vi "data_store.vi"(9 "Action":enum16{"set values", "get values"}(ring), 11 "number of elements":i32=10000) -> (1 "Variant":variant, 2 "array items":cluster{"name":string, "address":string}[](array[cluster]), 3 "names":string[](array[string]))   [LabVIEW 2018]
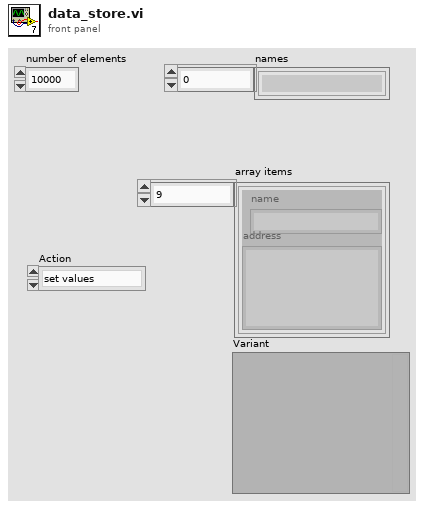
[diagram p1: front panel]
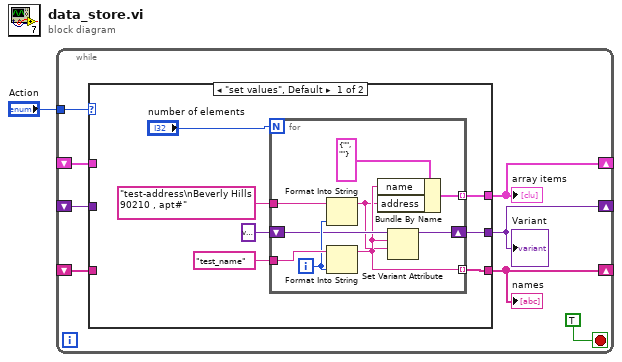
[diagram p0: block diagram]
diagram:
  n1 = while {
    shift-right: [w8] -> _
    shift-left: _ -> [w7]
    shift-right: [w4] -> _
    shift-left: _ -> [w6]
    tunnel: "Action" -> [w5]
    shift-right: [w3] -> _
    shift-left: _ -> [w2]
    stop <- TRUE stop-if-true
    n2 = case shown="\"set values\", Default" w5 {
      tunnel: [w13 w28] -> w8
      tunnel: [w12 w27] -> w4
      tunnel: w7 -> [_ w28]
      tunnel: w6 -> [_ w27]
      tunnel: [w10 w26] -> w3
      tunnel: w2 -> [_ w26]
      frame "set values", Default {
        n3 = for {
          N: "number of elements" -> [_]
          tunnel: "test_name" -> [w25]
          tunnel: "test-address\nBeverly Hills 90210 , apt#" -> [w23]
          tunnel: [w22] -> w12 mode=indexing
          tunnel: [w19] -> w13 mode=indexing
          shift-right: [w17] -> w10
          shift-left: variant -> [w20]
          i -> [w24]
          n4 = Format Into String(initial string=w23, w24) -> (resulting string=w18:string)  [unwired: 2 in, 1 out]
          n5 = Format Into String(initial string=w25, w24) -> (resulting string=w19:string)  [unwired: 2 in, 1 out]
          n6 = Bundle By Name(cluster=cluster{"name":string, "address":string} {"name"="", "address"=""} ("element"), "name"=w19, "address"=w18) -> (w22:cluster{"name":string, "address":string})
          n7 = Set Variant Attribute(Variant=w20, name=w19, value=w18) -> (Variant out=w17:variant)  [unwired: 1 in, 2 out]
        }
      }
      frame "get values" {
      }
    }
    "names" <- w8
    "array items" <- w4
    "Variant" <- w3
  }
